vi "13.vi"() -> (0 "Error Out":errorcluster)   [LabVIEW 2017, in "ErrorStructureDrawer-Tests.lvlib"]
uses:
  ErrorStructureDrawer-Tests.lvlib
panel:
  in  "asfasdfasdf":dbl
  in  "x 2":dbl
  out "x*y":dbl
  in  "x":dbl
  in  "y":dbl
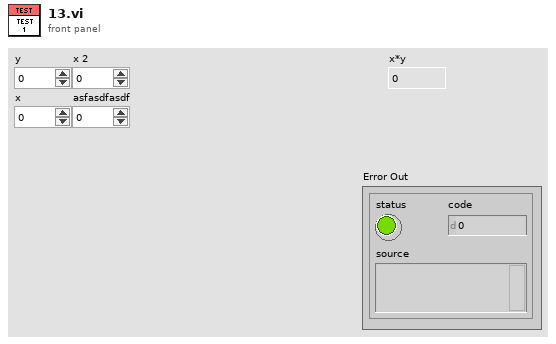
[diagram p1: front panel]
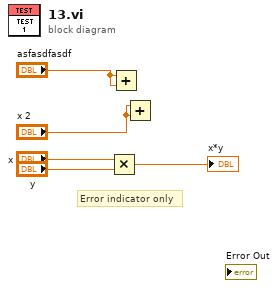
[diagram p0: block diagram]
diagram:
  # "Error indicator only"
  n1 = Multiply(x="x", y="y") -> (x*y=→"x*y":dbl)
  n2 = Add(x="asfasdfasdf", y="asfasdfasdf") -> ()  [unwired: 1 out]
  n3 = Add(x="x 2", y="x 2") -> ()  [unwired: 1 out]
